vi "Draw Circle (ARGB).vi"(5 "Thickness (Default: 1)":i32=1, 6 "OpenCV Line Type (Default LINE_8)":T4=enum."LINE_8", 7 "ARGB Colour":T2={"Alpha"=255, "RGB"=0}, 8 "error in (no error)":errorcluster, 9 "Radius":u16, 10 "Centre":T3, 11 "ARGB Image in":T1) -> (0 "error out":errorcluster, 3 "ARGB Image":T1)   [LabVIEW 2020, in "image.lvlib"]
doc: "Draw a circle at the specified centre-point with the given radius."
uses:
  image.lvlib
  Line Type.ctl
  common/Image Point (Integer).ctl
  ARGB Image.ctl
  ARGB Colour.ctl
  8336a1cf-e433-4bea-8080-376bdb783d4e.vi
  <vilib>/Utility/error.llb/Error Cluster From Error Code.vi
  common/common.lvlib
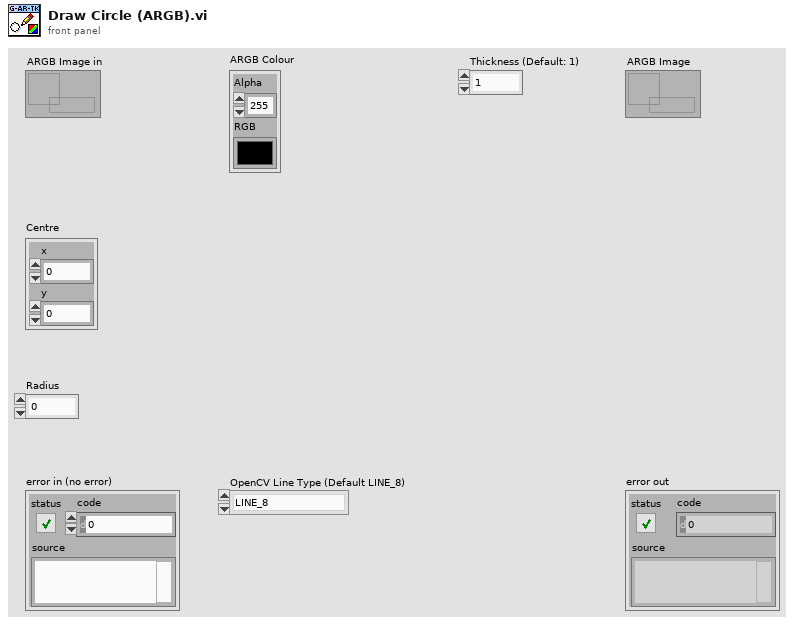
[diagram p1: front panel]
types:
  T1 = typedef "image.lvlib/ARGB Image.ctl" = refnum<data-value>
  T2 = typedef "image.lvlib/ARGB Colour.ctl" = cluster{"Alpha":u8, "RGB":u32}
  T3 = typedef "common.lvlib/Image Point (Integer).ctl" = cluster{"x":i32, "y":i32}
  T4 = typedef "image.lvlib/Line Type.ctl" = enum8{"FILLED", "LINE_4", "LINE_8", "LINE_AA"}
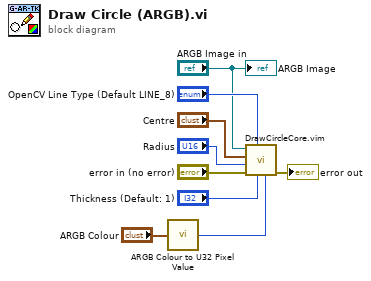
[diagram p0: block diagram]
diagram:
  n1 = call "ARGB Colour to U32 Pixel Value.vi"("ARGB Colour"="ARGB Colour") -> ("U32 Colour"=w2:u32)
  n2 = call "DrawCircleCore.vim"("Colour"=w2, "Thickness"="Thickness (Default: 1)", "OpenCV Line Type"="OpenCV Line Type (Default LINE_8)", "error in (no error)"="error in (no error)", "Radius"="Radius", "Centre"="Centre", "Src"="ARGB Image in") -> ("error out"=→"error out":errorcluster)  [unwired: 4 in]
  "ARGB Image" <- "ARGB Image in"
